vi "AudioStreamer.IsTrainer.vi"() -> (0 "trainer":bool)   [LabVIEW 2020]
uses:
  Typedefs/AudioStreamer.Globals.vi
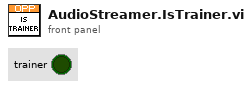
[diagram p1: front panel]
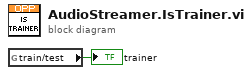
[diagram p0: block diagram]
diagram:
  n1 = global read "AudioStreamer.Globals.vi" "train/test"() -> (→"trainer":bool)
